vi "Principal-MSI.vi"() -> ()   [LabVIEW 2020]
panel:
  out "Decimal":dbl
  out "Azimut Solar":dbl(knob) scale=0.36..360.0
  out "Altura del Sol":dbl(knob) scale=-90.0..90.0
  in  "stop":bool
  out "Seg Solar":i32
  out "Min Solar":i32
  out "Hr Solar":i32
  out "Ecuación Tiempo":dbl
  out "DST":i32
  out "Fecha":string
  out "Ángulo Horario (w)":dbl(knob) scale=-180.0..180.0
  out "Declinación":dbl(knob) scale=23.45..-23.45
  out "Hora Solar":dbl
  out "Día del año (n)":dbl
  out "Hora Oficial":string
  out "Decimal":dbl
  in  "Segundos":i32
  in  "Minutos":i32
  in  "Grados":i32
  in  "Segundos":i32
  in  "Minutos":i32
  in  "Grados":i32
  # "INSTRUMENTACIÓN VIRTUAL"
  # "SEGUIDOR SOLAR"
  # "LATITUD NORTE (N)"
  # "LONGITUD OESTE (W)"
  # "N"
  # "S"
  # "N"
  # "UP"
  # "O"
  # "E"
  # "AZIMUT SOLAR"
  # "ELEVACIÓN"
  # "S"
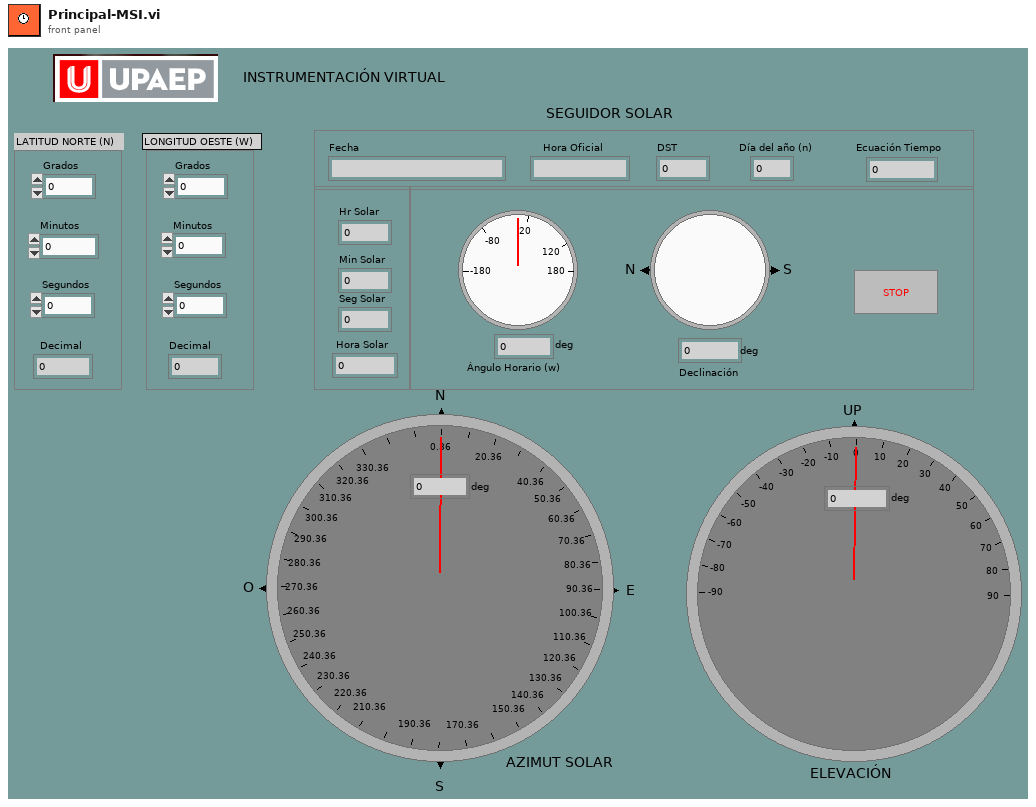
[diagram p1: front panel]
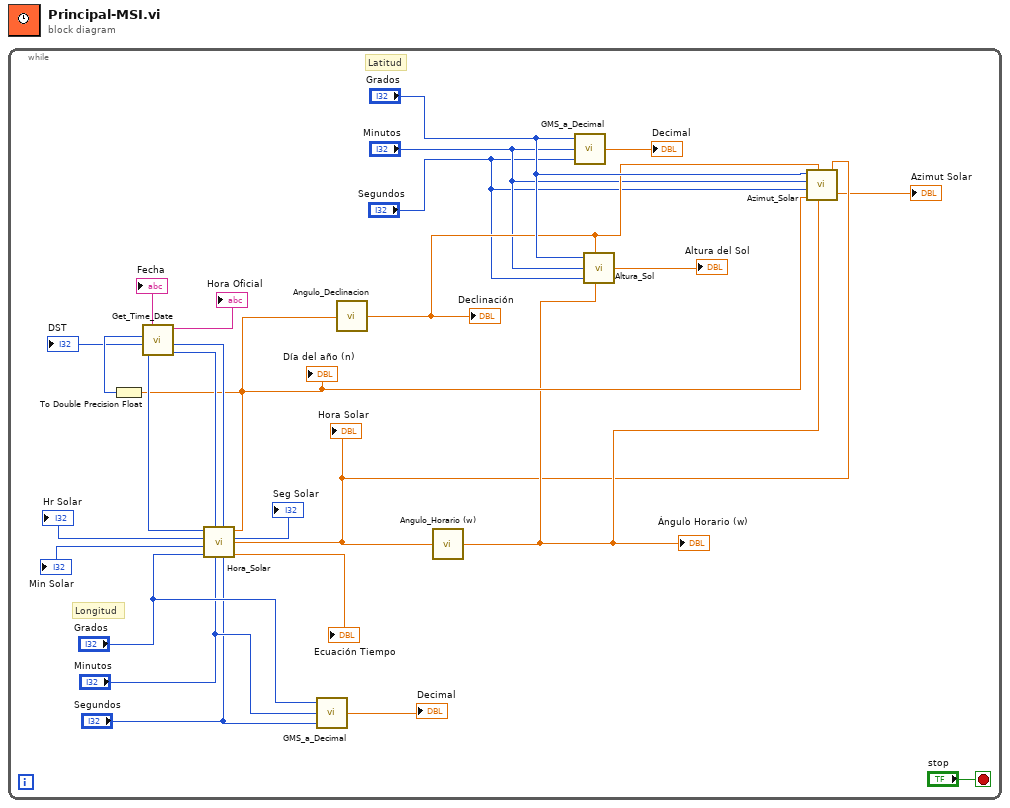
[diagram p0: block diagram]
diagram:
  n1 = while {
    stop <- "stop" stop-if-true
    # "Longitud"
    # "Latitud"
    n2 = call "Get_Time_Date.vi"() -> ("minute"=w21:i32, "second"=w22:i32, "time string"=→"Hora Oficial":string, "hour"=w23:i32, "DST"=→"DST":i32, "day of year"=w24:i32, "date string"=→"Fecha":string)  [unwired: 1 out]
    n3 = To Double Precision Float(number=w24) -> (double precision float=w11:dbl)
    "Día del año (n)" <- w11
    n4 = call "Hora_Solar.vi"("Grados"="Grados", "Min"="Minutos", "Seg"="Segundos", "Hora Oficial"=w23, "Min Oficial"=w21, "Seg Oficial"=w22, "Día del año (n)"=w11) -> ("Eq. Tiempo"=→"Ecuación Tiempo":dbl, "Min Solar"=→"Min Solar":i32, "Hora Solar"=w8:dbl, "Hr Solar"=→"Hr Solar":i32, "Seg Solar"=→"Seg Solar":i32)
    "Hora Solar" <- w8
    n5 = call "GMS_a_Decimal.vi"("Segundos"="Segundos", "Minutos"="Minutos", "Grados"="Grados") -> ("Decimal"=→"Decimal":dbl)
    n6 = call "Angulo_Declinacion.vi"("n"=w11) -> ("Declinación"=w9:dbl)
    "Declinación" <- w9
    n7 = call "Angulo_Horario (w).vi"("Hora Solar"=w8) -> ("Ángulo Horario (w)"=w10:dbl)
    "Ángulo Horario (w)" <- w10
    n8 = call "GMS_a_Decimal.vi"("Segundos"="Segundos", "Minutos"="Minutos", "Grados"="Grados") -> ("Decimal"=→"Decimal":dbl)
    n9 = call "Altura_Sol.vi"("Grados"="Grados", "Declinación"=w9, "Minutos"="Minutos", "Segundos"="Segundos", "Ángulo Horario"=w10) -> ("Altura del Sol"=→"Altura del Sol":dbl)
    n10 = call "Azimut_Solar.vi"("Hora Solar"=w8, "Angulo Horario"=w10, "Declinacion"=w9, "n"=w11, "Segundos"="Segundos", "Minutos"="Minutos", "Grados"="Grados") -> ("Azimut Solar"=→"Azimut Solar":dbl)
  }
